vi "Configure Display View.vi"(8 "error in (no error)":errorcluster, 9 "Screen Layout (0: Standard View)":i32(ring) items=["Standard View", "Large Text", "Large Graph", "CH1/CH2"], 10 "Displayed Channel (1: 1)":i32(ring)=1 items=["1"=1, "2"=2], 11 "VISA resource name":refnum<visa-resource-name>) -> (0 "error out":errorcluster, 3 "VISA resource name out":refnum<visa-resource-name>)   [LabVIEW 2015, in "Agilent 3352X Series.lvlib"]
doc: "Configures the screen layout, and specifies the displayed channel on a two-channel instrument.\n\n<b>Note</b>:\nThis VI is only applicable for 33611A, 33612A, 33621A and 33622A models."
uses:
  <instrlib>/Agilent 3352X Series/Agilent 3352X Series.lvlib
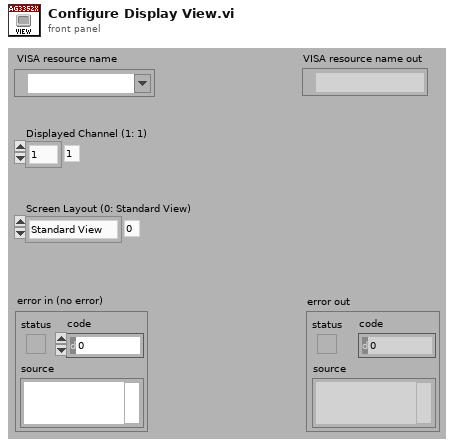
[diagram p1: front panel]
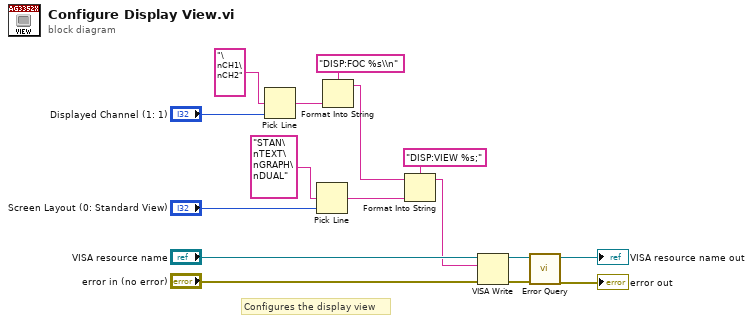
[diagram p0: block diagram]
diagram:
  # "Configures the display view"
  n1 = Pick Line(multi-line string="\nCH1\nCH2", line index="Displayed Channel (1: 1)") -> (output string=w2:string)  [unwired: 1 out]
  n2 = Pick Line(multi-line string="STAN\nTEXT\nGRAPH\nDUAL", line index="Screen Layout (0: Standard View)") -> (output string=w7:string)  [unwired: 1 out]
  n3 = Format Into String(format string="DISP:FOC %s\\n", w2) -> (resulting string=w1:string)  [unwired: 2 in, 1 out]
  n4 = Format Into String(format string="DISP:VIEW %s;", initial string=w1, w7) -> (resulting string=w6:string)  [unwired: 1 in, 1 out]
  n5 = VISA Write(VISA resource name="VISA resource name", write buffer=w6, error in (no error)="error in (no error)") -> (VISA resource name out=w16:refnum<visa-resource-name>, error out=w15:errorcluster)  [unwired: 1 out]
  n6 = call <instrlib>:"Error Query.vi"("error in (no error)"=w15, "VISA resource name"=w16) -> ("error out"=→"error out":errorcluster, "VISA resource name out"=→"VISA resource name out":refnum<visa-resource-name>)  [unwired: 8 out]
